vi "HWAsync Cmd END Dialog.vi"(8 "error in (no error)":errorcluster, 10 "Msg in":string, 11 "Message Queue":refnum<queue>) -> (0 "error out":errorcluster, 2 "Msg out":string)   [LabVIEW 2014]
uses:
  APIs/Message Queue/Message Cluster.ctl
  APIs/Message Queue/Enqueue Message (Single).vi
  APIs/Message Queue/WINFAS 2 Message Queue.lvlib
panel:
  in  "Action Buttons":T1
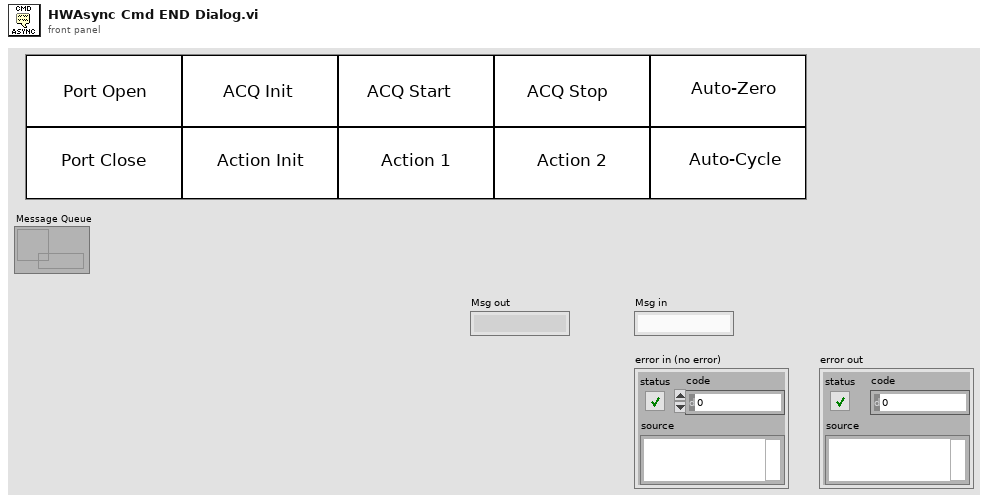
[diagram p1: front panel]
types:
  T1 = cluster{"Port Open":bool, "Port Close":bool, "ACQ Init":bool, "ACQ Start":bool, "ACQ Stop":bool, "Action Init":bool, "Action 1":bool, "Action 2":bool, "Auto-Zero":bool, "Auto-Cycle":bool}
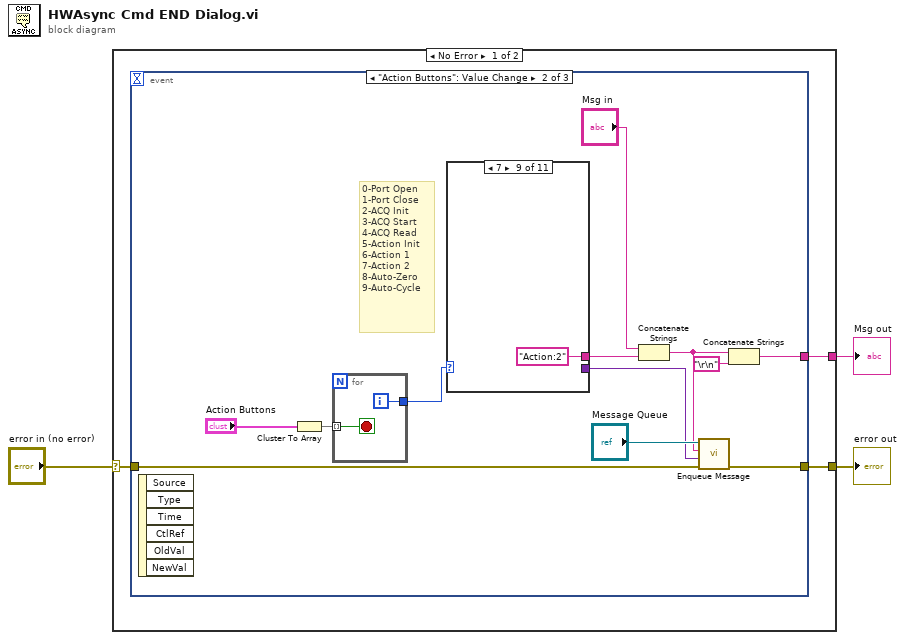
[diagram p0: block diagram]
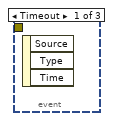
[diagram p2: hidden frame]
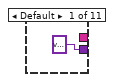
[diagram p3: hidden frame]
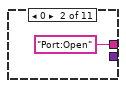
[diagram p4: hidden frame]
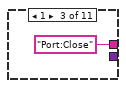
[diagram p5: hidden frame]
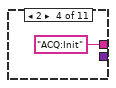
[diagram p6: hidden frame]
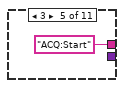
[diagram p7: hidden frame]
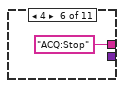
[diagram p8: hidden frame]
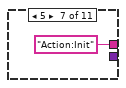
[diagram p9: hidden frame]
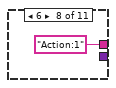
[diagram p10: hidden frame]
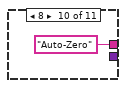
[diagram p11: hidden frame]
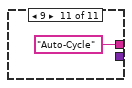
[diagram p12: hidden frame]
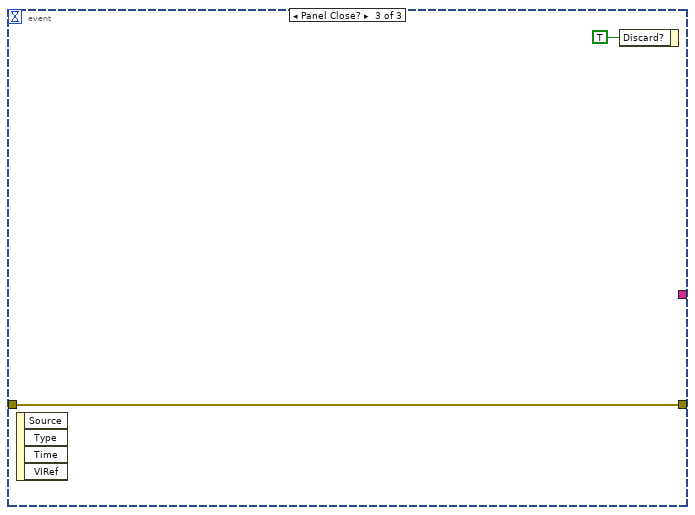
[diagram p13: hidden frame]
diagram:
  n1 = case shown="No Error" "error in (no error)" {
    selector: "error in (no error)" -> [w6 w34]
    tunnel: [w5 w34] -> w2
    tunnel: [w4 _] -> w1
    frame No Error {
      n2 = event shown="[1] \"Action Buttons\": Value Change" {
        selector: _ -> [_ _ _]
        dyn-events: _ -> [_ _ _]
        timeout: _ -> [_ _ _]
        tunnel: w6 -> [_ w12 w32]
        tunnel: [_ w11 w32] -> w5
        tunnel: [_ w7 _] -> w4
        event Timeout {
          n3 = event-data() -> ()  [unwired: 1 in, 3 out]
        }
        event "Action Buttons": Value Change {
          # "0-Port Open\n1-Port Close\n2-ACQ Init\n3-ACQ Start\n4-ACQ Read\n5-Action Init\n6-Action 1\n7-Action 2\n8-Auto-Zero\n9-Auto-Cycle"
          n4 = event-data() -> ()  [unwired: 1 in, 6 out]
          n5 = Cluster To Array(cluster="Action Buttons") -> (array=w17:bool[])
          n6 = for {
            tunnel: w17 -> [w20] mode=indexing
            tunnel: [w19] -> w16
            i -> [w19]
            stop <- w20 stop-if-true
          }
          n7 = case shown="7" w16 {
            tunnel: [_ "Port:Open" "Port:Close" "ACQ:Init" "ACQ:Start" "ACQ:Stop" "Action:Init" "Action:1" "Action:2" "Auto-Zero" "Auto-Cycle"] -> w15
            tunnel: [variant _ _ _ _ _ _ _ _ _ _] -> w10
            frame Default {
            }
            frame 0 {
            }
            frame 1 {
            }
            frame 2 {
            }
            frame 3 {
            }
            frame 4 {
            }
            frame 5 {
            }
            frame 6 {
            }
            frame 7 {
            }
            frame 8 {
            }
            frame 9 {
            }
          }
          n8 = Concatenate Strings("Msg in", w15) -> (w8:string)
          n9 = call-poly "Enqueue Message.vi"("error in (no error)"=w12, "Message Data"=w10, "Message"=w8, "Message Queue"="Message Queue") -> ("error out"=w11:errorcluster)  [unwired: 6 in, 1 out]
          n10 = Concatenate Strings(w8, "\r\n") -> (w7:string)
        }
        event Panel Close? {
          n11 = event-data() -> ()  [unwired: 1 in, 4 out]
          n12 = event-data("Discard?"=TRUE) -> ()  [unwired: 1 in, 1 out]
        }
      }
    }
    frame Error {
    }
  }
  "error out" <- w2
  "Msg out" <- w1
